vi "loadM300MachineStatus.vi"(10 "name or relative path":string="M420_LSTR機台狀況(早)_12月.xls", 11 "template (empty)":path=path "c:/m300") -> ()   [LabVIEW 2012]
uses:
  <vilib>/addons/database/Auxilliary.llb/DB Tools Cursor Type.ctl
  <vilib>/Utility/NIReport.llb/NI_report.lvclass
  <vilib>/addons/database/Connection.llb/DB Tools Open Connec (Path).vi
  <vilib>/addons/database/Connection.llb/Conn Execute.vi
  <vilib>/addons/database/Recordset.llb/Rec Destroy - Connection.vi
  <vilib>/addons/_office/excel.llb/Excel Get Data (str).vi
  <vilib>/Utility/NIReport.llb/Excel/NI_Excel.lvclass
  <vilib>/addons/_office/NI_ReportGenerationToolkit.lvlib
  <vilib>/addons/database/NI_Database_API.lvlib
panel:
  out "error out 5":errorcluster
  out "error out 3":errorcluster
  out "error out 4":errorcluster
  out "concatenated string":string
  out "output cluster":T1
  out "after substring":string
  out "error out":errorcluster
  out "x > y?":bool
  out "s? t:f":string
  in  "Cluster 2":T1
  in  "array 2":string[][](array[string])
  out "Numeric":i32
  out "x+y 2":i32
  out "array":string[](array[string])
  out "data 3":string
  in  "start (0, 0) 3":cluster{"start row":i32, "start column":i32}
  out "data 2":string
  in  "start (0, 0) 2":cluster{"start row":i32, "start column":i32}
  out "data":string
  in  "start (0, 0)":cluster{"start row":i32, "start column":i32}
  out "x+y":i32
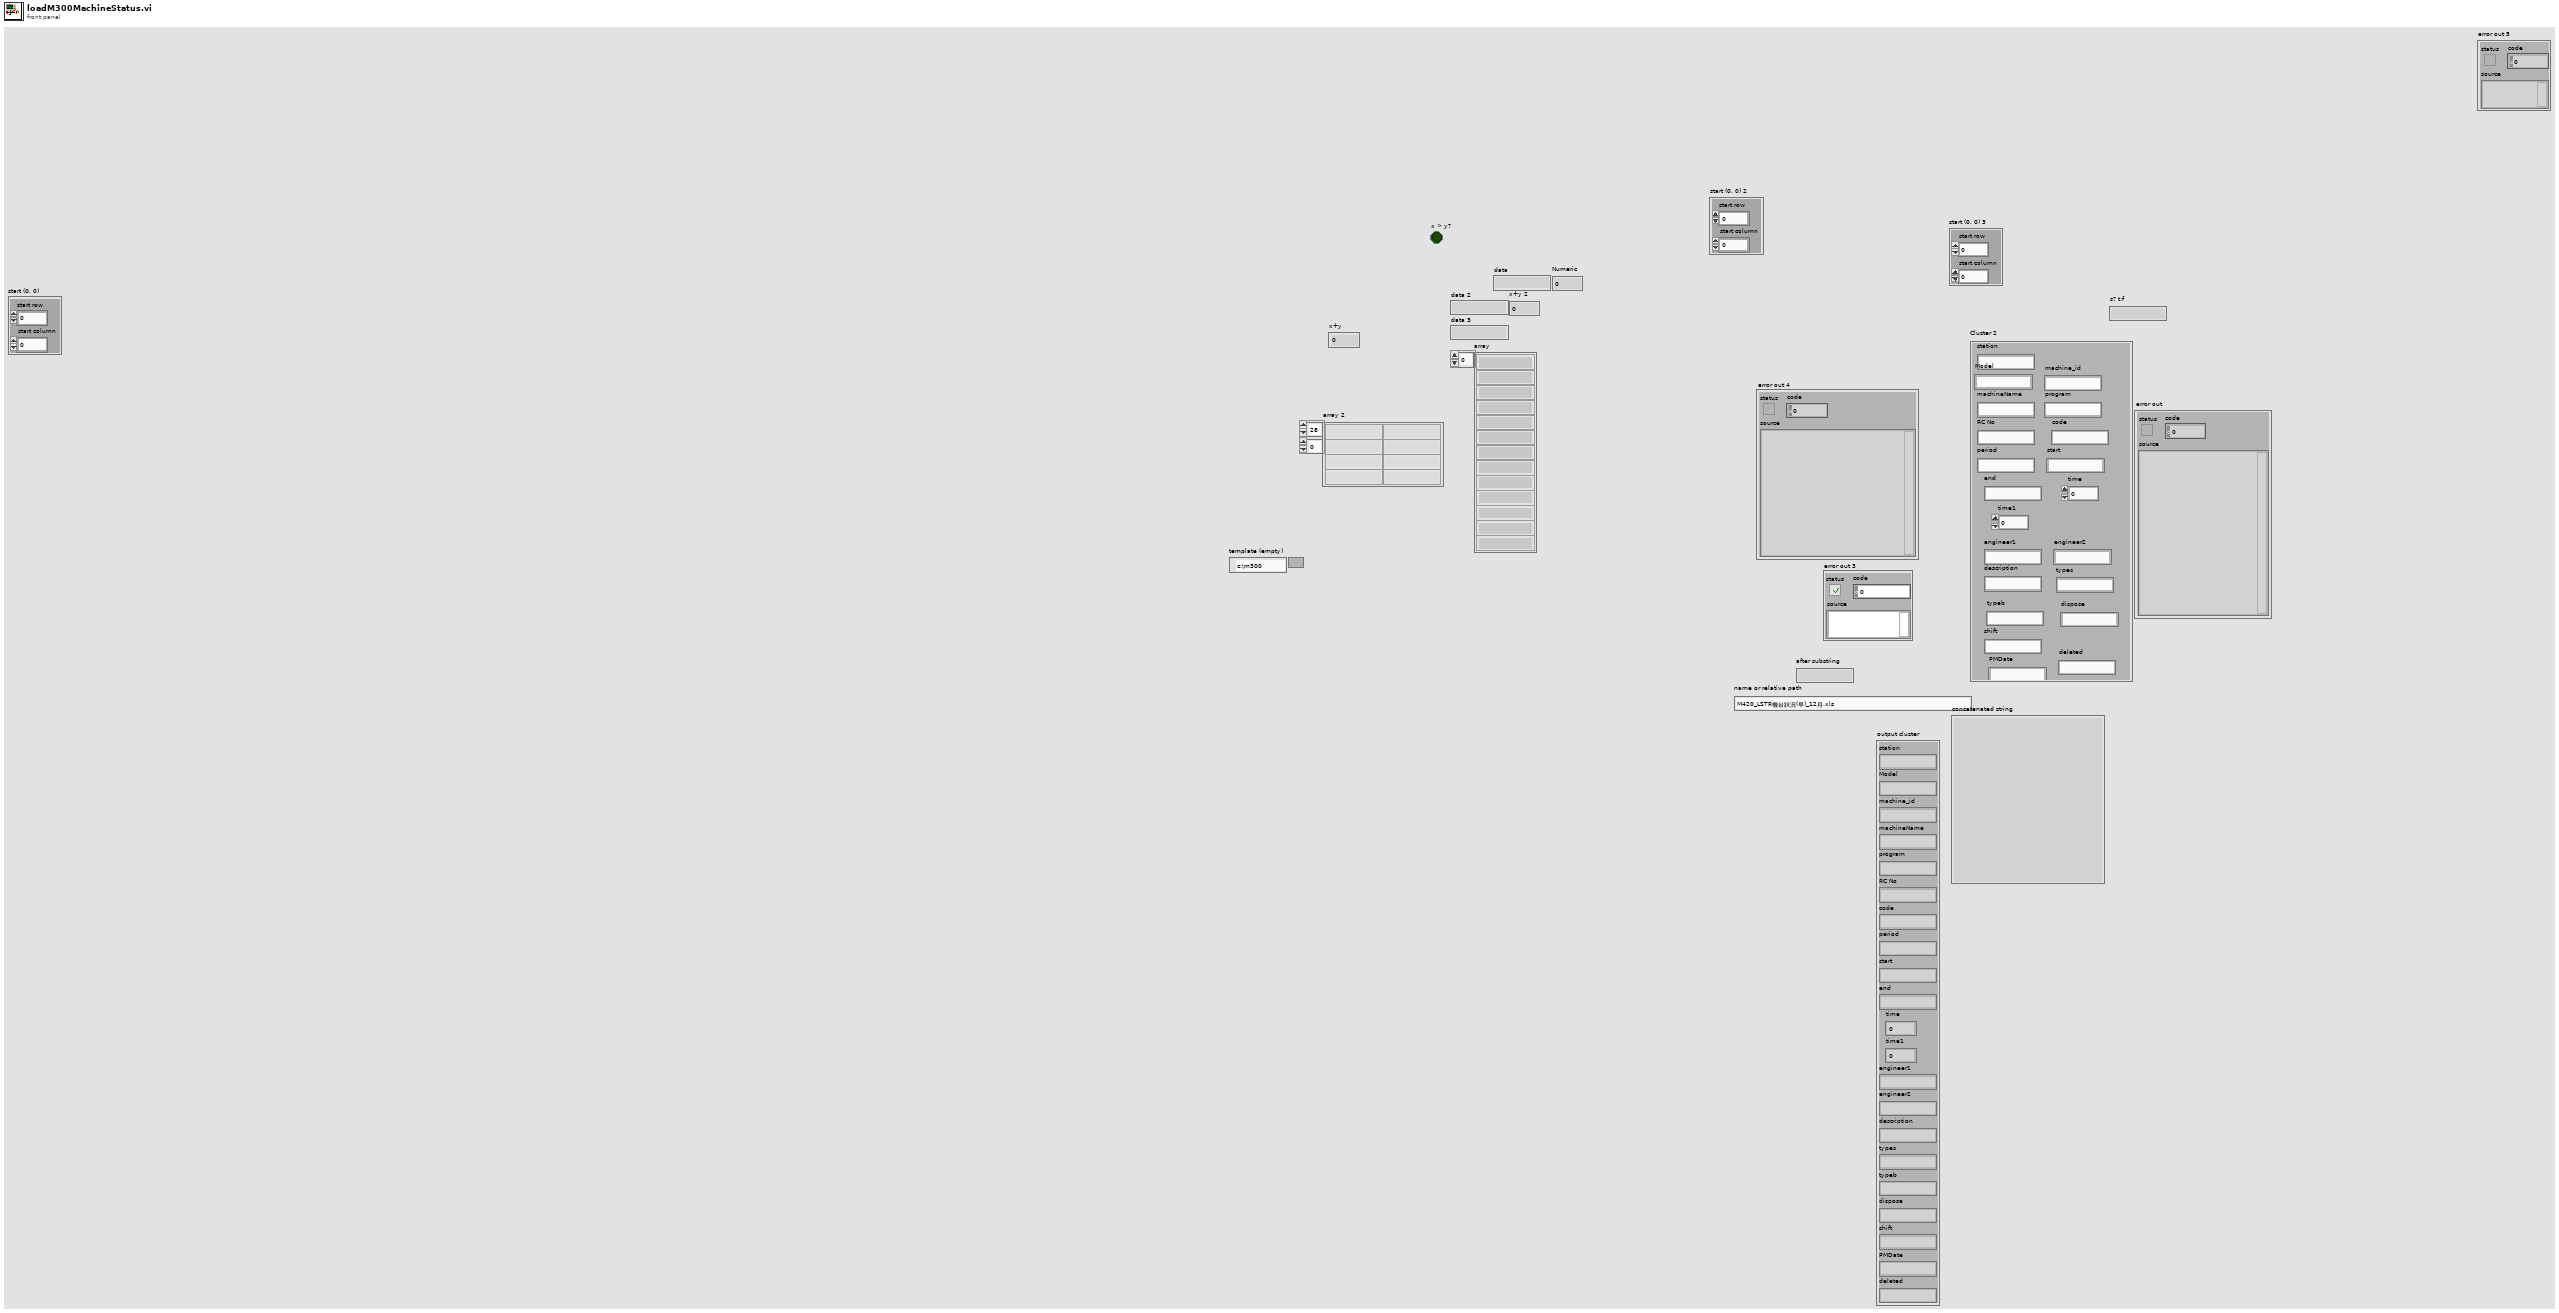
[diagram p1: front panel]
types:
  T1 = cluster{"station":string, "Model":string, "machine_id":string, "machineName":string, "program":string, "RC No":string, "code":string, "period":string, "start":string, "end":string, "time":dbl, "time1":dbl, "engineer1":string, "engineer2":string, "description":string, "types":string, "typeb":string, "dispose":string, "shift":string, "PMDate":string, "deleted":string}
  T2 = enum16{"Standard Report", "HTML", "Word", "Excel"}
  T3 = typedef "NI_Database_API.lvlib/Conn ObjectReference.ctl" = refnum<k1>
  T4 = typedef "NI_Database_API.lvlib/DB Tools Cursor Type.ctl" = enum16{"forward-only", "keyset", "dynamic", "static"}
  T5 = typedef "NI_Database_API.lvlib/Rec ObjectReference.ctl" = refnum<k1>
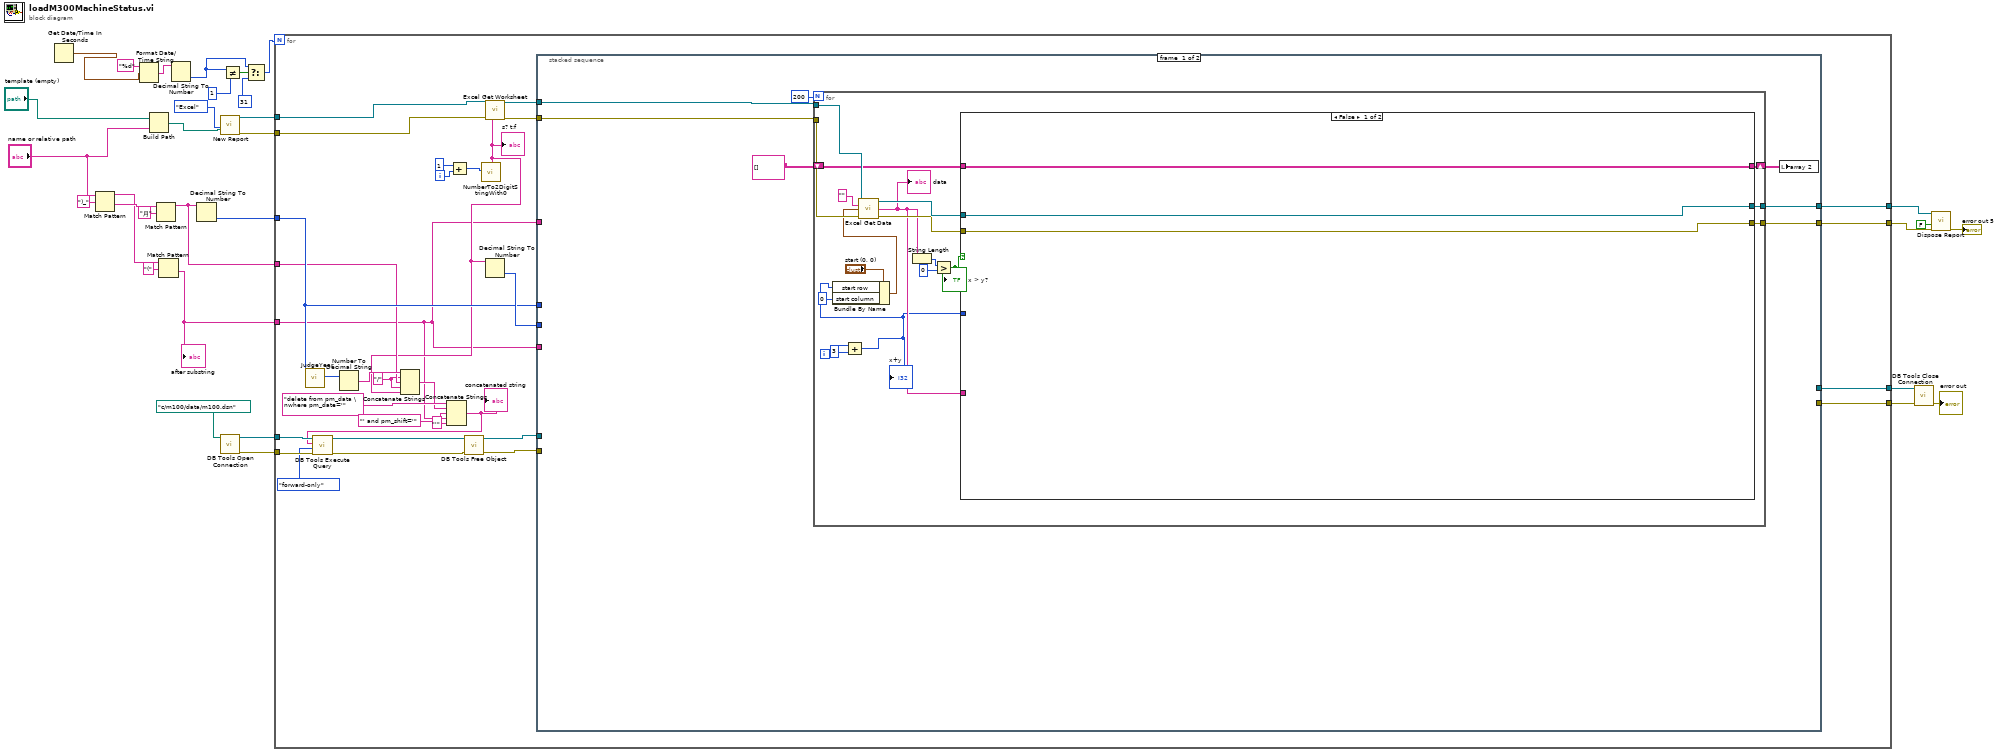
[diagram p0: block diagram]
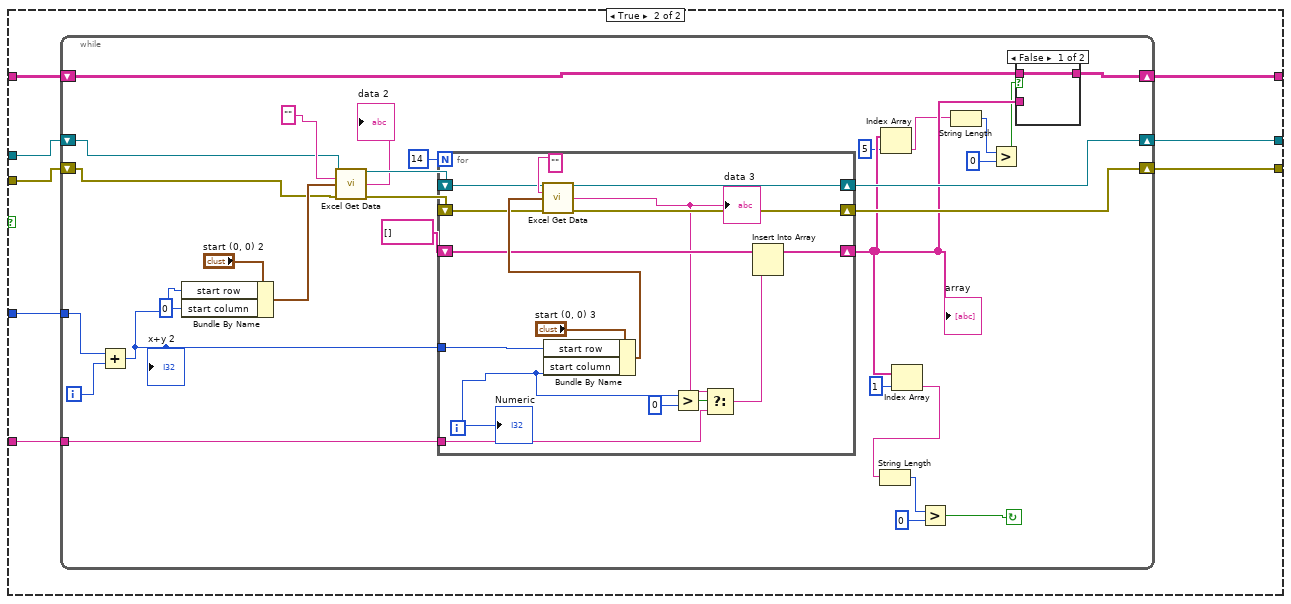
[diagram p2: hidden frame]
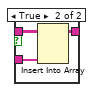
[diagram p3: hidden frame]
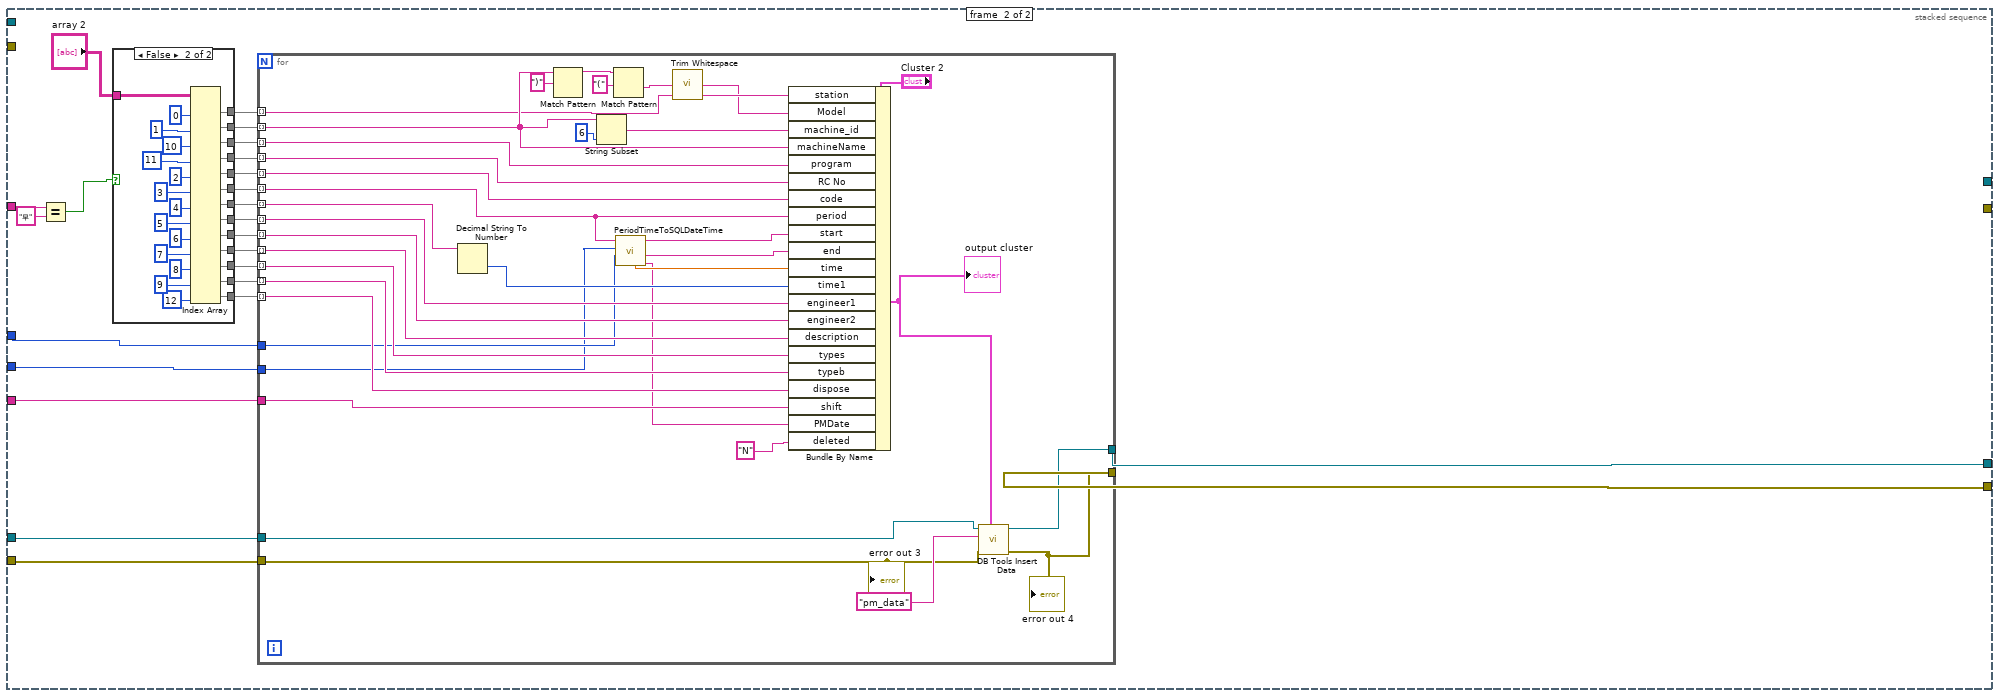
[diagram p4: hidden frame]
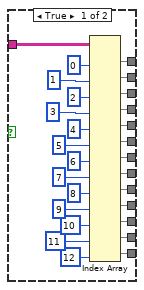
[diagram p5: hidden frame]
diagram:
  n1 = Get Date/Time In Seconds() -> (seconds since 1Jan1904=w21:timestamp)
  n2 = Match Pattern(string="name or relative path", regular expression=")_") -> (before substring=w25:string, after substring=w32:string)  [unwired: 1 in, 2 out]
  n3 = Format Date/Time String(time format string (%c)="%d", seconds (now)=w21) -> (date/time string=w22:string)  [unwired: 1 in]
  n4 = Build Path(base path="template (empty)", name or relative path="name or relative path") -> (appended path=w14:path)
  n5 = Match Pattern(string=w32, regular expression="月") -> (before substring=w9:string)  [unwired: 1 in, 3 out]
  n6 = Match Pattern(string=w25, regular expression="(") -> (after substring=w24:string)  [unwired: 1 in, 3 out]
  "after substring" <- w24
  n7 = Decimal String To Number(string=w22) -> (number=w17:i32)  [unwired: 2 in, 1 out]
  n8 = Decimal String To Number(string=w9) -> (number=w27:i32)  [unwired: 2 in, 1 out]
  n9 = call <vilib>:"New Report.vi"("report type"=T2."Excel" ("Report Type"), "template (empty)"=w14) -> ("report out"=w13:refnum<class "NI_report.lvclass">, "error out"=w12:errorcluster)  [unwired: 12 in]
  n10 = call-poly <vilib>:"DB Tools Open Connection.vi"("connection information"=path "c:/m100/data/m100.dsn") -> ("error out"=w10:errorcluster, "connection reference"=w11:T3)  [unwired: 7 in]
  n11 = Not Equal?(x=w17, y=1) -> (x != y?=w19:bool)
  n12 = Select(t=w17, s=w19, f=31) -> (s? t:f=w1:i32)
  n13 = for {
    N: w1 -> [_]
    tunnel: w27 -> [w56]
    tunnel: w24 -> [w36]
    tunnel: w13 -> [w58]
    tunnel: w12 -> [w57]
    tunnel: w11 -> [w38]
    tunnel: w10 -> [w40]
    tunnel: w9 -> [w53]
    tunnel: [w48] -> w7
    tunnel: [w47] -> w6
    tunnel: [w34] -> w3
    tunnel: [w33] -> w2
    i -> [w61]
    w52 = "/" ("string")
    n14 = call "JudgeYear.vi"("DataMonth"=w56) -> ("DataYear"=w55:i32)  [unwired: 10 in]
    n15 = Number To Decimal String(number=w55) -> (decimal integer string=w54:string)  [unwired: 1 in]
    n16 = Add(x=1, y=w61) -> (x+y=w45:i32)
    n17 = call "NumberTo2DigitStringWith0.vi"("number"=w45) -> ("s? t:f"=w46:string)  [unwired: 10 in]
    "s? t:f" <- w46
    n18 = Concatenate Strings(w54, w52, w53, w52, w46) -> (w50:string)
    n19 = Concatenate Strings("delete from pm_data \nwhere pm_date='" ("string"), w50, "' and pm_shift='" ("string"), w36, "'" ("string")) -> (w37:string)
    "concatenated string" <- w37
    n20 = call-poly <vilib>:"DB Tools Execute Query.vi"("error in (no error)"=w40, "cursor type"=DB_Tools_Cursor_Type."forward-only", "SQL query"=w37, "connection reference"=w38) -> ("error out"=w41:errorcluster, "recordset reference"=w42:T5)  [unwired: 4 in]
    n21 = call-poly <vilib>:"DB Tools Free Object.vi"("error in (no error)"=w41, "recordset reference"=w42) -> ("error out"=w43:errorcluster, "connection reference"=w44:T3)  [unwired: 8 in]
    n22 = call <vilib>:"Excel Get Worksheet.vi"("report in"=w58, "error in (no error)"=w57, "name (\"\")"=w46) -> ("report out"=w63:refnum<class "NI_report.lvclass">, "error out"=w62:errorcluster)  [unwired: 11 in]
    n23 = Decimal String To Number(string=w46) -> (number=w59:i32)  [unwired: 2 in, 1 out]
    n24 = stacked-sequence {
      tunnel: w63 -> [w67 _]
      tunnel: w62 -> [w66 _]
      tunnel: w56 -> [_ w160]
      tunnel: w59 -> [_ w159]
      tunnel: w36 -> [_ w158]
      tunnel: w36 -> [_ w157]
      tunnel: w44 -> [_ w154]
      tunnel: w43 -> [_ w153]
      tunnel: [_ w152] -> w48
      tunnel: [_ w151] -> w47
      tunnel: [w65 _] -> w34
      tunnel: [w64 _] -> w33
      frame #0 {
        n25 = for {
          N: 200 -> [_]
          tunnel: w67 -> [w89]
          tunnel: w66 -> [w88]
          shift-right: [w76] -> w69
          shift-left: string[][] [] ("array") -> [w75]
          tunnel: [w72] -> w65
          tunnel: [w71] -> w64
          i -> [w84]
          n26 = Add(x=w84, y=3) -> (x+y=w73:i32)
          "x+y" <- w73
          n27 = Bundle By Name(cluster="start (0, 0)", "start row"=w73, "start column"=0) -> (w85:cluster{"start row":i32, "start column":i32})
          n28 = call-poly <vilib>:"Excel Get Data.vi"("report in"=w89, "data type"="", "start (0, 0)"=w85, "error in (no error)"=w88) -> ("report out"=w81:refnum<class "NI_report.lvclass">, "data"=w74:string, "error out"=w80:errorcluster)  [unwired: 9 in]
          "data" <- w74
          n29 = String Length(string=w74) -> (length=w79:i32)
          n30 = Greater?(x=w79, y=0) -> (0:w77:bool)
          "x > y?" <- w77
          n31 = case shown="False" w77 {
            tunnel: w73 -> [_ w100]
            tunnel: w81 -> [w91 w99]
            tunnel: w80 -> [w90 w98]
            tunnel: [w92 w97] -> w76
            tunnel: w75 -> [w92 w96]
            tunnel: w74 -> [_ w95]
            tunnel: [w91 w94] -> w72
            tunnel: [w90 w93] -> w71
            frame False {
            }
            frame True {
              n32 = while {
                tunnel: w100 -> [w129]
                shift-right: [w119] -> w97
                shift-left: w96 -> [w118]
                shift-right: [w117] -> w94
                shift-left: w99 -> [w115]
                shift-right: [w116] -> w93
                shift-left: w98 -> [w114]
                tunnel: w95 -> [w101]
                i -> [w128]
                stop <- w109 continue-if-true
                n33 = Add(x=w129, y=w128) -> (x+y=w122:i32)
                "x+y 2" <- w122
                n34 = Bundle By Name(cluster="start (0, 0) 2", "start row"=w122, "start column"=0) -> (w127:cluster{"start row":i32, "start column":i32})
                n35 = call-poly <vilib>:"Excel Get Data.vi"("report in"=w115, "data type"="", "start (0, 0)"=w127, "error in (no error)"=w114) -> ("report out"=w123:refnum<class "NI_report.lvclass">, "data"=→"data 2":string, "error out"=w124:errorcluster)  [unwired: 9 in]
                n36 = for {
                  N: 14 -> [_]
                  shift-right: [w147] -> w117
                  shift-left: w123 -> [w145]
                  shift-right: [w146] -> w116
                  shift-left: w124 -> [w144]
                  tunnel: w122 -> [w141]
                  shift-right: [w143] -> w108
                  shift-left: string[] [] ("array") -> [w142]
                  tunnel: w101 -> [w135]
                  i -> [w140]
                  n37 = Bundle By Name(cluster="start (0, 0) 3", "start row"=w141, "start column"=w140) -> (w149:cluster{"start row":i32, "start column":i32})
                  n38 = call-poly <vilib>:"Excel Get Data.vi"("report in"=w145, "data type"="", "start (0, 0)"=w149, "error in (no error)"=w144) -> ("report out"=w147:refnum<class "NI_report.lvclass">, "data"=w137:string, "error out"=w146:errorcluster)  [unwired: 9 in]
                  "data 3" <- w137
                  n39 = Greater?(x=w140, y=0) -> (0:w138:bool)
                  n40 = Select(t=w137, s=w138, f=w135) -> (s? t:f=w136:string)
                  n41 = Insert Into Array(array=w142, new element=w136) -> (w143:string[])  [unwired: 1 in]
                  "Numeric" <- w140
                }
                "array" <- w108
                n42 = Index Array(array=w108, index=5) -> (element=w104:string)
                n43 = Index Array(array=w108, index=1) -> (element=w110:string)
                n44 = String Length(string=w110) -> (length=w113:i32)
                n45 = Greater?(x=w113, y=0) -> (0:w109:bool)
                n46 = String Length(string=w104) -> (length=w106:i32)
                n47 = Greater?(x=w106, y=0) -> (0:w103:bool)
                n48 = case shown="False" w103 {
                  tunnel: [w131 w134] -> w119
                  tunnel: w118 -> [w131 w133]
                  tunnel: w108 -> [_ w132]
                  frame False {
                  }
                  frame True {
                    n49 = Insert Into Array(array=w133, new element=w132) -> (w134:string[][])  [unwired: 2 in]
                  }
                }
              }
            }
          }
        }
        n50 = local write "array 2"(w69) -> ()
      }
      frame #1 {
        n51 = Equal?(x=w157, y="早") -> (x = y?=w155:bool)
        n52 = case shown="False" w155 {
          tunnel: "array 2" -> [w201 w228]
          tunnel: [w200 w227] -> w173
          tunnel: [w199 w226] -> w172
          tunnel: [w198 w225] -> w171
          tunnel: [w197 w224] -> w170
          tunnel: [w196 w223] -> w169
          tunnel: [w195 w222] -> w168
          tunnel: [w194 w221] -> w167
          tunnel: [w193 w220] -> w166
          tunnel: [w192 w219] -> w165
          tunnel: [w191 w218] -> w164
          tunnel: [w190 w217] -> w163
          tunnel: [w189 w216] -> w162
          tunnel: [w188 w215] -> w161
          frame True {
            n53 = Index Array(array=w201, index (col) #1=0 ("disabled index (col)"), index (col) #2=1 ("index (col)"), index (col) #3=2 ("index (col)"), index (col) #4=3 ("index (col)"), index (col) #5=4 ("index (col)"), index (col) #6=5 ("index (col)"), index (col) #7=6 ("index (col)"), index (col) #8=7 ("index (col)"), index (col) #9=8 ("index (col)"), index (col) #10=9 ("index (col)"), index (col) #11=10 ("index (col)"), index (col) #12=11 ("index (col)"), index (col) #13=12 ("index (col)")) -> (element #1=w200:string[], element #2=w199:string[], element #3=w198:string[], element #4=w197:string[], element #5=w196:string[], element #6=w195:string[], element #7=w194:string[], element #8=w193:string[], element #9=w192:string[], element #10=w191:string[], element #11=w190:string[], element #12=w189:string[], element #13=w188:string[])  [unwired: 13 in]
          }
          frame False {
            n54 = Index Array(array=w228, index (col) #1=0 ("disabled index (col)"), index (col) #2=1 ("index (col)"), index (col) #3=10 ("index (col)"), index (col) #4=11 ("index (col)"), index (col) #5=2 ("index (col)"), index (col) #6=3 ("index (col)"), index (col) #7=4 ("index (col)"), index (col) #8=5 ("index (col)"), index (col) #9=6 ("index (col)"), index (col) #10=7 ("index (col)"), index (col) #11=8 ("index (col)"), index (col) #12=9 ("index (col)"), index (col) #13=12 ("index (col)")) -> (element #1=w227:string[], element #2=w226:string[], element #3=w225:string[], element #4=w224:string[], element #5=w223:string[], element #6=w222:string[], element #7=w221:string[], element #8=w220:string[], element #9=w219:string[], element #10=w218:string[], element #11=w217:string[], element #12=w216:string[], element #13=w215:string[])  [unwired: 13 in]
          }
        }
        n55 = for {
          tunnel: w173 -> [w234] mode=indexing
          tunnel: w172 -> [w235] mode=indexing
          tunnel: w171 -> [w262] mode=indexing
          tunnel: w170 -> [w261] mode=indexing
          tunnel: w169 -> [w260] mode=indexing
          tunnel: w168 -> [w242] mode=indexing
          tunnel: w167 -> [w258] mode=indexing
          tunnel: w166 -> [w257] mode=indexing
          tunnel: w165 -> [w256] mode=indexing
          tunnel: w164 -> [w255] mode=indexing
          tunnel: w163 -> [w254] mode=indexing
          tunnel: w162 -> [w253] mode=indexing
          tunnel: w161 -> [w252] mode=indexing
          tunnel: [w247] -> w152
          tunnel: [w246] -> w151
          tunnel: w160 -> [w244]
          tunnel: w159 -> [w243]
          tunnel: w158 -> [w241]
          tunnel: w154 -> [w230]
          tunnel: w153 -> [w229]
          n56 = Decimal String To Number(string=w258) -> (number=w251:i32)  [unwired: 2 in, 1 out]
          n57 = Match Pattern(string=w235, regular expression=")") -> (before substring=w236:string)  [unwired: 1 in, 3 out]
          n58 = String Subset(string=w235, length (rest)=6 ("length (rest)")) -> (substring=w263:string)  [unwired: 1 in]
          n59 = Match Pattern(string=w236, regular expression="(") -> (after substring=w232:string)  [unwired: 1 in, 3 out]
          n60 = call "PeriodTimeToSQLDateTime.vi"("day"=w243, "Month"=w244, "string"=w242) -> ("StingDate"=w239:string, "SQLDatetime2"=w249:string, "SQLDateTime1"=w250:string, "Period(M)"=w248:dbl)  [unwired: 5 in]
          n61 = call <vilib>:"Trim Whitespace.vi"("string"=w232) -> ("trimmed string"=w233:string)  [unwired: 1 in]
          n62 = Bundle By Name(cluster="Cluster 2", "station"=w234, "Model"=w233, "machine_id"=w263, "machineName"=w235, "program"=w262, "RC No"=w261, "code"=w260, "period"=w242, "start"=w250, "end"=w249, "time"=w248, "time1"=w251, "engineer1"=w257, "engineer2"=w256, "description"=w255, "types"=w254, "typeb"=w253, "dispose"=w252, "shift"=w241, "PMDate"=w239, "deleted"="N") -> (w245:T1)
          "output cluster" <- w245
          n63 = call <vilib>:"DB Tools Insert Data.vi"("data"=w245, "error in (no error)"=w229, "table"="pm_data", "connection reference"=w230) -> ("error out"=w246:errorcluster, "connection reference out"=w247:T3)  [unwired: 6 in]
          "error out 4" <- w246
          "error out 3" <- w229
        }
      }
    }
  }
  n64 = call <vilib>:"DB Tools Close Connection.vi"("error in (no error)"=w6, "connection reference"=w7) -> ("error out"=→"error out":errorcluster)  [unwired: 5 in]
  n65 = call-dynamic "Dispose Report.vi"("report in"=w3, "save changes? (F)"=FALSE, "error in (no error)"=w2) -> ("error out"=→"error out 5":errorcluster)  [unwired: 12 in]
